vi "prepCI2_tt.vi"   [LabVIEW 2013]
uses:
  <vilib>/DAQmx/create/channels.llb/DAQmx Create Channel (CI-Count Edges).vi
  <vilib>/DAQmx/configure/timing.llb/DAQmx Timing (Sample Clock).vi
  <resource>/objmgr/daqmx.rc
types:
  T1 = cluster{"CH1 AI":tag, "CH1 CI":tag, "CH2 AI":tag, "CH2 CI":tag, "AI X":tag, "AI Y":tag, "AO X-Y":tag, "CH1ST":bool, "CH2ST":bool, "Sigcase":i16, "StageS":i32, "StageL":i32, "data dir":path, "Vp":tag, "Ip":tag, "AO CWlaser":tag, "AO VtoP":tag, "shutter":tag, "488":tag, "532":tag, "640":tag, "LT marker":tag, "image OD":u16, "contour OD":u16, "point OD":u16}
  T2 = typedef "LVRectTypeDef.ctl" = cluster{"Left":i16, "Top":i16, "Right":i16, "Bottom":i16}
  T3 = cluster{"Xpixels":i32, "Vxminref":dbl, "Vxmaxref":dbl, "P":dbl, "Ypixels":i32, "Vyminref":dbl, "Vymaxref":dbl, "srate":sgl, "sAOxy":i32, "timeout":dbl, "type":string, "date":string, "time":string, "Colormap":u16, "Drawing Mode":u16, "Scanning Mode":u16, "square pixels":bool, "square matrix":bool, "Xpixels Img":i32, "Vx-min Img":dbl, "VX-max Img":dbl, "Ypixels Img":i32, "Vy-min Img":dbl, "Vy-max Img ":dbl, "Angle Img":dbl, "autoshutter":bool, "finite":bool, "cont":bool, "wavdet":bool, "measpoints":i32, "avpp":i32, "bufferAO":i32, "bufferAI":i32, "CH1":bool, "CH2":bool, "X":bool, "Y":bool, "Ip":bool, "Vp":bool, "starttick":u32, "waveform":path, "Vx-ref":dbl, "Vy-ref":dbl, "refreshrate":dbl, "refreshbuffer":i32, "tt_cycles":i32, "motorref":refnum<k7>, "mirrorswitch":refnum<k7>, "sample mode":i32, "maxbufferAI":i32, "sampletreshold":dbl, "srateAODO":sgl, "bin":sgl, "Pel":sgl, "Angle draw":dbl, "srate Img":sgl, "ROIimg_plotbounds":T2, "auto OD":bool, "ODfilt":u16, "reset AO_DO":bool}
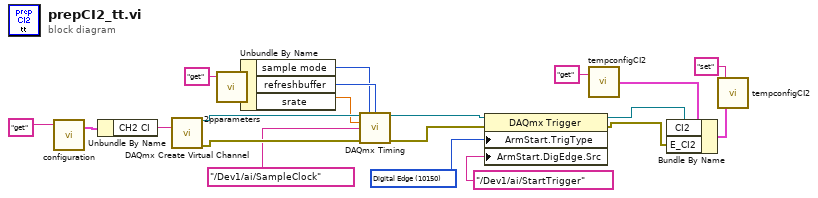
[diagram p0: block diagram]
diagram:
  w20 = 10150 items=["Digital Edge"=10150, "None"=10230] ("ArmStart.TrigType")
  n1 = call "configuration.vi"("command"="get") -> ("config out"=w15:T1)  [unwired: 2 in, 1 out]
  n2 = Unbundle By Name(w15) -> ("CH2 CI"=w14:tag)
  n3 = call-poly <vilib>:"DAQmx Create Virtual Channel.vi"("counter"=w14) -> ("task out"=w17:refnum<k21>, "error out"=w18:errorcluster)  [unwired: 13 in]
  n4 = call "2pparameters.vi"("command"="get") -> ("Params out"=w11:T3)  [unwired: 1 in]
  n5 = Unbundle By Name(w11) -> ("sample mode"=w1:i32, "refreshbuffer"=w9:i32, "srate"=w6:sgl)
  n6 = call-poly <vilib>:"DAQmx Timing.vi"("task/channels in"=w17, "sample mode"=w1, "samples per channel"=w9, "rate"=w6, "source"=tag "/Dev1/ai/SampleClock", "error in"=w18) -> ("task out"=w12:refnum<k21>, "error out"=w21:errorcluster)  [unwired: 8 in]
  n7 = property class="DAQmx Trigger"(reference=w12, error in=w21, "ArmStart.TrigType"=w20, "ArmStart.DigEdge.Src"=tag "/Dev1/ai/StartTrigger") -> (reference out=w4:refnum<k21>, error out=w3:errorcluster)
  n8 = call "tempconfigCI2.vi"("command"="get") -> ("Temp Config out"=w5:cluster{"CI2":refnum<k21>, "E_CI2":errorcluster})  [unwired: 1 in]
  n9 = Bundle By Name(cluster=w5, "CI2"=w4, "E_CI2"=w3) -> (w2:cluster{"CI2":refnum<k21>, "E_CI2":errorcluster})
  n10 = call "tempconfigCI2.vi"("Temp Config in"=w2, "command"="set") -> ()  [unwired: 1 out]
